vi "C to F.vi"(1 "Degrees C":dbl) -> (0 "Degrees F":dbl)   [LabVIEW 2020]
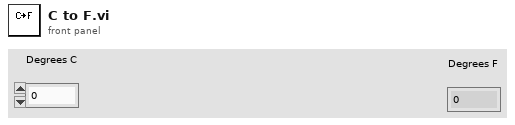
[diagram p1: front panel]
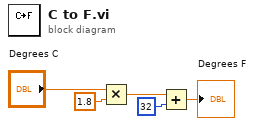
[diagram p0: block diagram]
diagram:
  n1 = Multiply(x="Degrees C", y=1.8) -> (x*y=w2:dbl)
  n2 = Add(x=w2, y=32) -> (x+y=→"Degrees F":dbl)
